vi "Save.vi"(8 "error in":errorcluster, 11 "state in":T1) -> (0 "error out":errorcluster, 3 "state out":T1)   [LabVIEW 2013, in "Advanced Configuration Tool.lvlib"]
doc: "This VI calls the Repo Save VI passing the current Path. Updating the unsaved changes flag if the save is succesfull."
uses:
  Advanced Configuration Tool.lvlib
  Controls/StateCluster.ctl
  Configuration Framework/Repository/NISE_CEF_Repository.lvclass
  Configuration Framework/Node/NodeRef.ctl
  Configuration Framework/Node/NISE_CEF_Node.lvclass
  Configuration Framework/Node/UserEventRef.ctl
  Configuration Framework/Controls/EventCluster.ctl
  Configuration Framework/NISE_CEF_TreeControl.lvlib
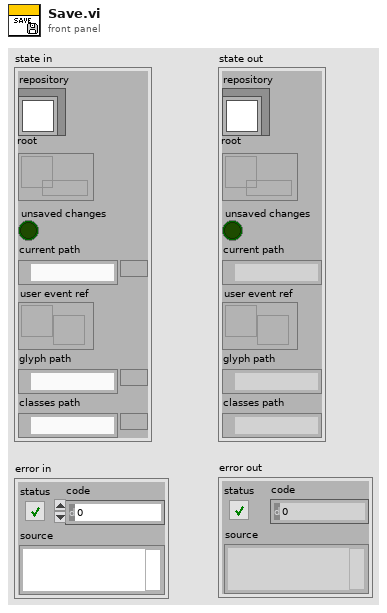
[diagram p1: front panel]
types:
  T1 = typedef "Advanced Configuration Tool.lvlib/StateCluster.ctl" = cluster{"repository":refnum<class "NISE_CEF_Repository.lvclass">, "root":T2, "unsaved changes":bool, "current path":path, "user event ref":T3, "glyph path":path, "classes path":path}
  T2 = typedef "NISE_CEF_Node.lvclass/NodeRef.ctl" = refnum<data-value>
  T3 = typedef "NISE_CEF_Node.lvclass/UserEventRef.ctl" = refnum<user-event>
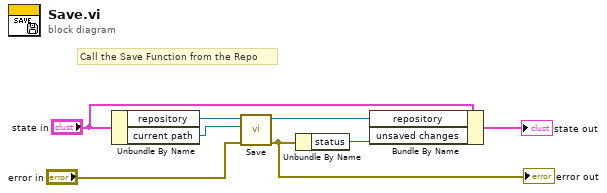
[diagram p0: block diagram]
diagram:
  # "Call the Save Function from the Repo"
  n1 = Unbundle By Name("state in") -> ("repository"=w8:refnum<class "NISE_CEF_Repository.lvclass">, "current path"=w2:path)
  n2 = call-dynamic "Save.vi"("error in"="error in", "file path"=w2, "repository in"=w8) -> ("error out"=w4:errorcluster, "repository out"=w1:refnum<class "NISE_CEF_Repository.lvclass">)  [unwired: 7 in]
  "error out" <- w4
  n3 = Unbundle By Name(w4) -> ("status"=w3:bool)
  n4 = Bundle By Name(cluster="state in", "repository"=w1, "unsaved changes"=w3) -> (→"state out":T1)
